vi "cRIO_8maze_controls_v3_nodoors.vi"() -> ()   [LabVIEW 2019]
panel:
  in  "Servo wait (ms)":u32=1000
  in  "Servo enable":bool
  in  "NO LEDs":bool
  in  "servo2PWM_R":dbl=3.4 format="%#_13g"
  in  "PWM initial":dbl[](array[numeric])=[9.5, 8.1, 5.1, 5.6]
  in  "MDServoPWM_R":dbl[](array[numeric])=[5.2, 5.45]
  in  "MDServoPWM_L":dbl[](array[numeric])=[5.2, 5.45]
  in  "No Milk":bool
  in  "Repeat sound":bool
  in  "Initialize":bool=TRUE
  in  "Air puff time":u32=1000
  in  "MD time (ms)":i32=3000
  out "Direction array":bool[](array[boolean])=[TRUE, FALSE, FALSE, TRUE, FALSE, TRUE, TRUE, FALSE, TRUE, FALSE, FALSE, TRUE, FALSE, TRUE, FALSE, FALSE, TRUE, FALSE, TRUE, TRUE, FALSE, TRUE, FALSE, FALSE, TRUE, FALSE, TRUE, TRUE, FALSE, TRUE, FALSE, FALSE, TRUE, FALSE, TRUE, TRUE, FALSE, TRUE, FALSE, FALSE, TRUE, FALSE, TRUE, TRUE, FALSE, TRUE, FALSE, FALSE, TRUE]
  out "Seq update":i32
  in  "Loop seq.":dbl
  out "All BBR":bool
  out "BB3_R":bool
  out "BB2_R":bool
  out "BB1_L":bool
  out "All BBL":bool
  out "BB3_L":bool
  out "BB2_L":bool
  out "BB1_R":bool
  out "Right":bool=TRUE
  in  "Sound":bool
  in  "AIR":bool
  out "Left":bool=TRUE
  in  "MD_R":bool
  in  "MD_L":bool
  in  "LED_R":bool
  in  "LED_L":bool
  in  "PWM rate":dbl[](array[numeric])=[0.1, 0.1, 0.1, 0.1]
  out "appended array":bool[](array[boolean])
  in  "PWM positions":dbl[](array[numeric])=[4.5, 3.4, 5.1, 5.8]
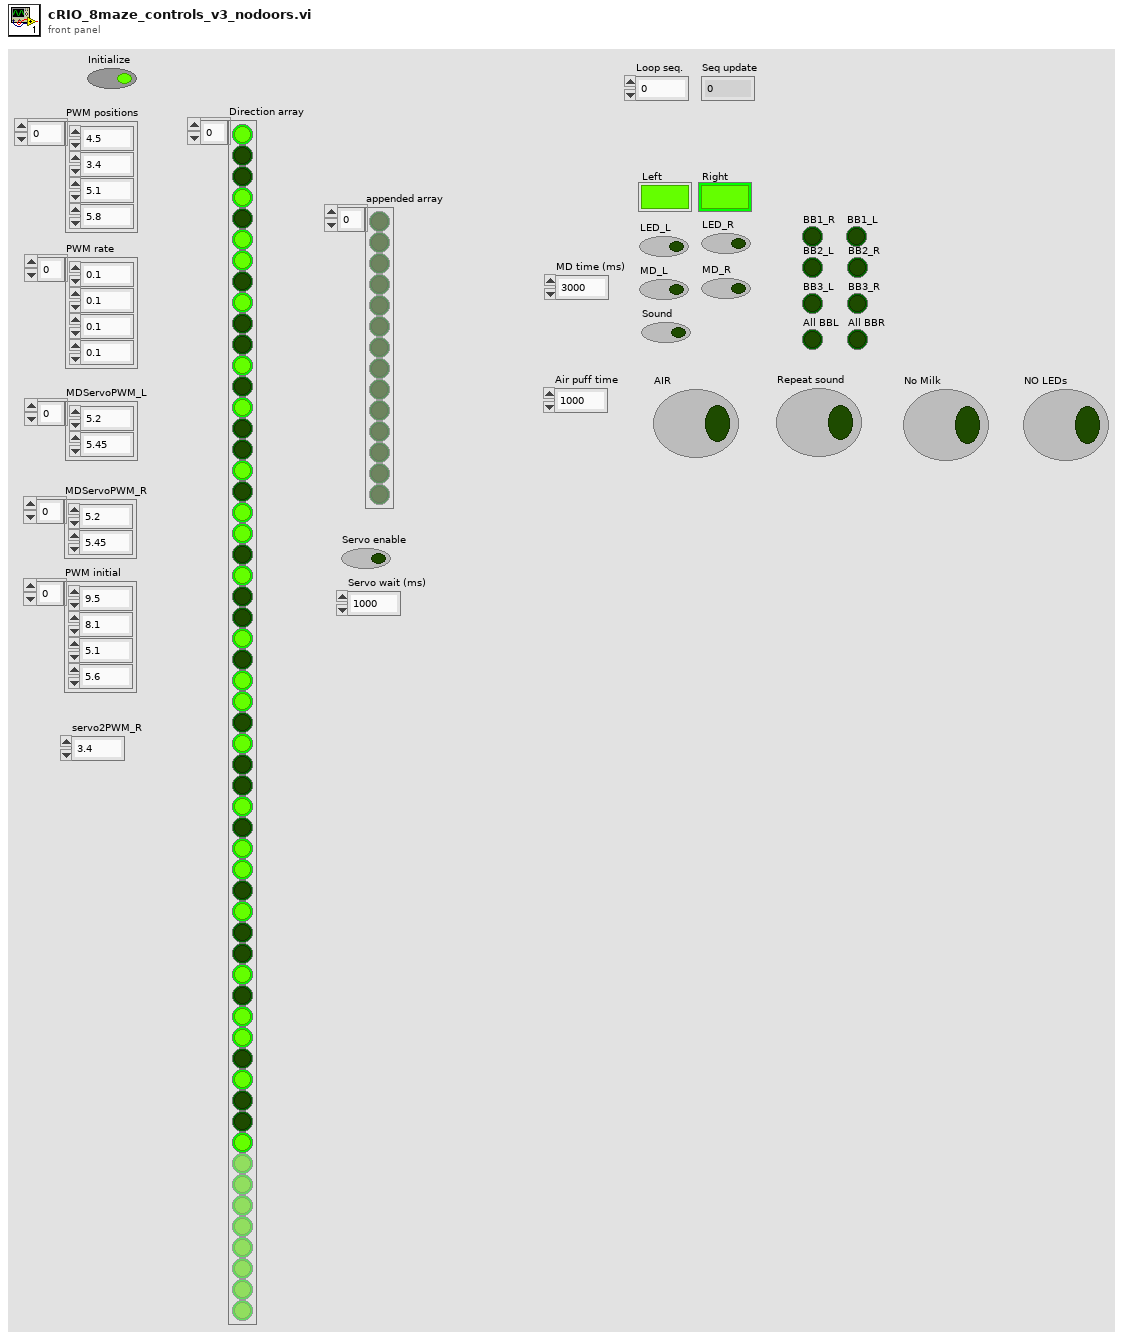
[diagram p1: front panel]
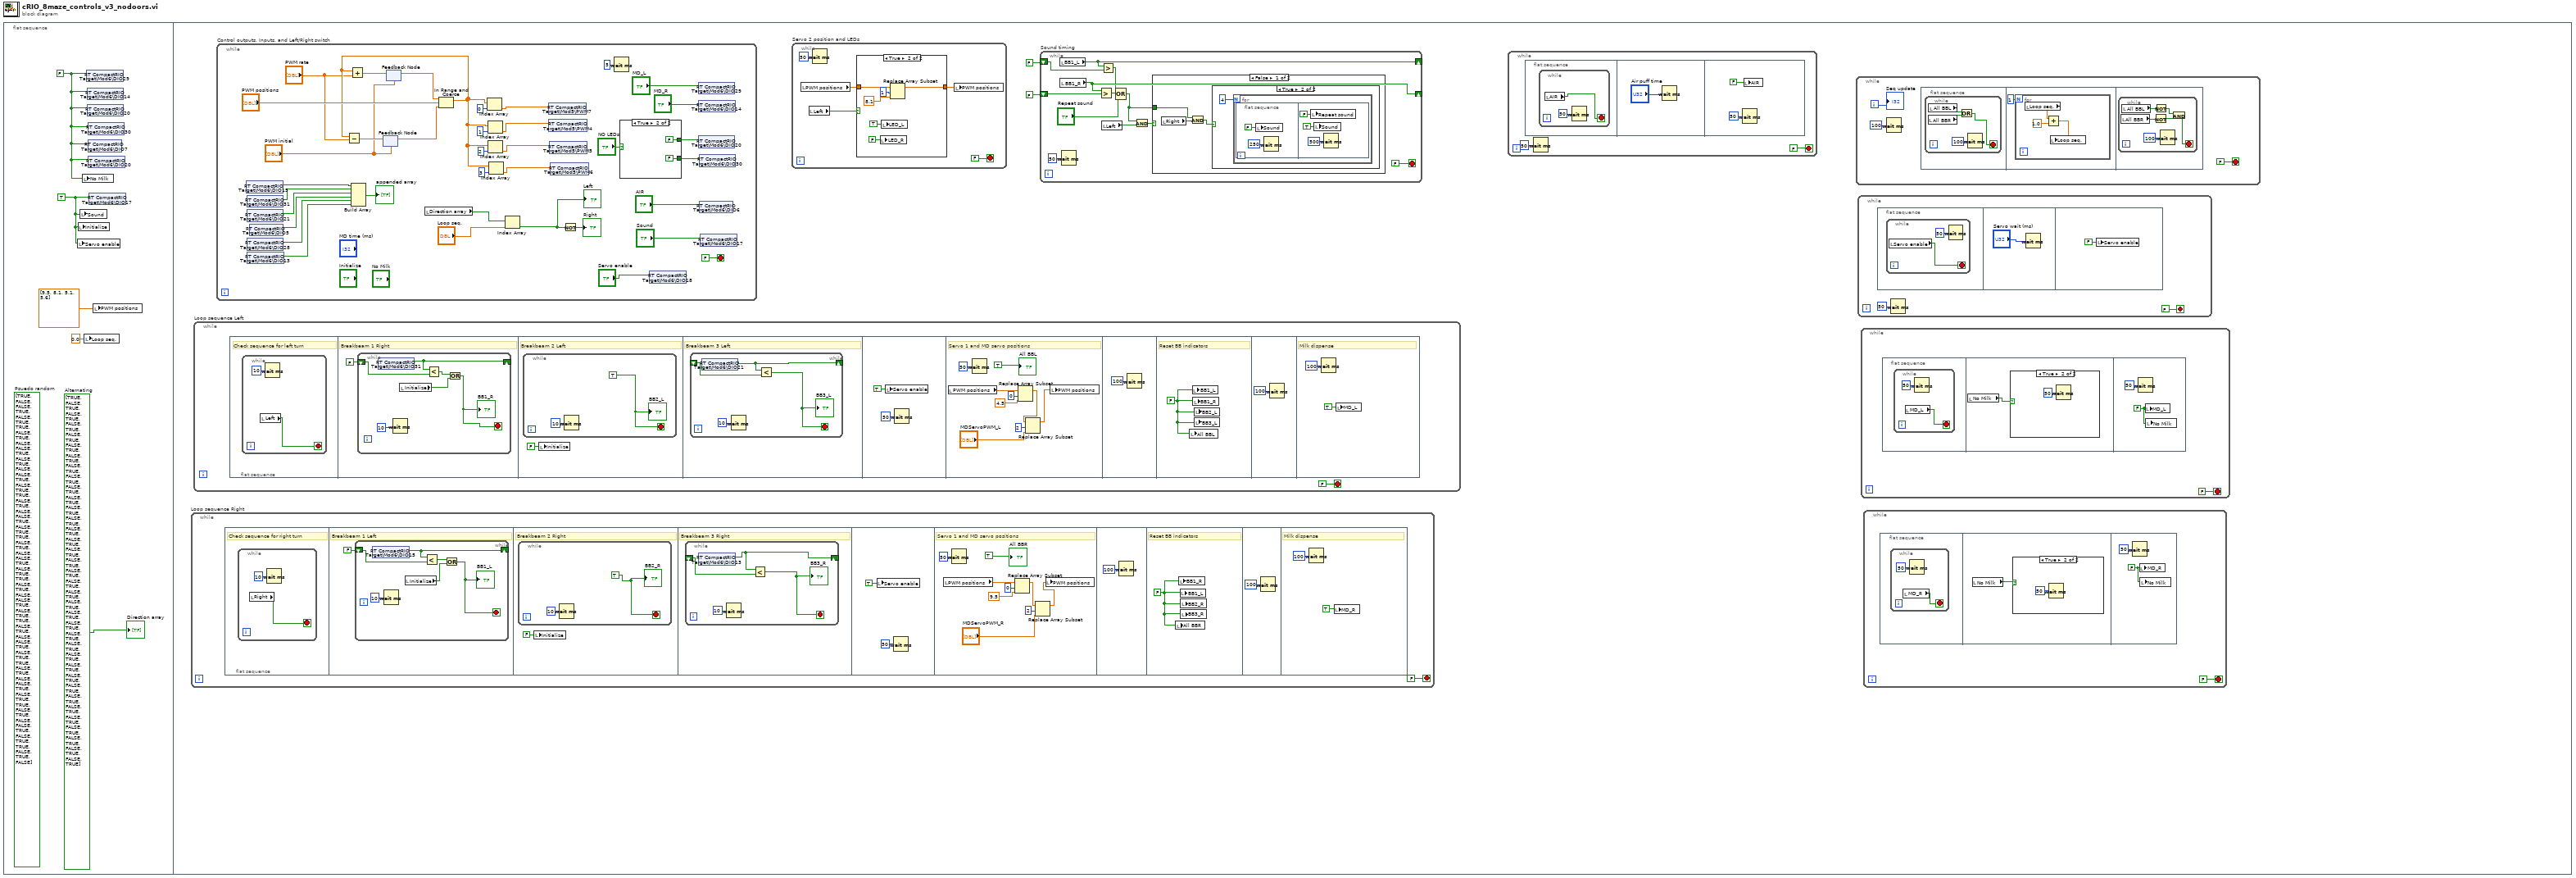
[diagram p0: block diagram]
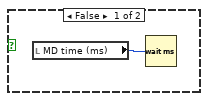
[diagram p2: hidden frame]
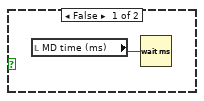
[diagram p3: hidden frame]
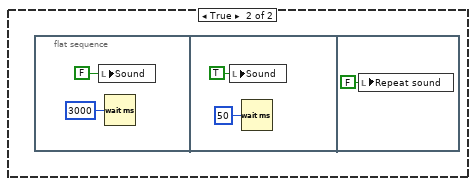
[diagram p5: hidden frame]
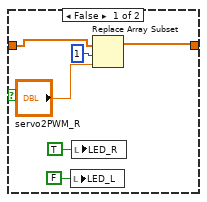
[diagram p6: hidden frame]
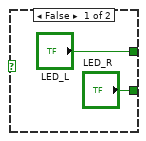
[diagram p7: hidden frame]
diagram:
  n1 = flat-sequence {
    frame #0 {
      w3 = bool[] [TRUE, FALSE, TRUE, FALSE, TRUE, FALSE, TRUE, FALSE, TRUE, FALSE, TRUE, FALSE, TRUE, FALSE, TRUE, FALSE, TRUE, FALSE, TRUE, FALSE, TRUE, FALSE, TRUE, FALSE, TRUE, FALSE, TRUE, FALSE, TRUE, FALSE, TRUE, FALSE, TRUE, FALSE, TRUE, FALSE, TRUE, FALSE, TRUE, FALSE, TRUE, FALSE, TRUE, FALSE, TRUE, FALSE, TRUE, FALSE, TRUE, FALSE, TRUE, FALSE, TRUE, FALSE, TRUE, FALSE, TRUE, FALSE, TRUE, FALSE, TRUE, FALSE, TRUE, FALSE, TRUE, FALSE, TRUE, FALSE, TRUE, FALSE, TRUE]  # Alternating
      (unwired) bool[] [TRUE, FALSE, FALSE, TRUE, FALSE, TRUE, TRUE, FALSE, TRUE, FALSE, FALSE, TRUE, FALSE, TRUE, FALSE, FALSE, TRUE, FALSE, TRUE, TRUE, FALSE, TRUE, FALSE, FALSE, TRUE, FALSE, TRUE, TRUE, FALSE, TRUE, FALSE, FALSE, TRUE, FALSE, TRUE, TRUE, FALSE, TRUE, FALSE, FALSE, TRUE, FALSE, TRUE, TRUE, FALSE, TRUE, FALSE, FALSE, TRUE, FALSE, TRUE, TRUE, FALSE, TRUE, FALSE, FALSE, TRUE, FALSE, TRUE, TRUE, FALSE, TRUE, FALSE, FALSE, TRUE, FALSE, TRUE, TRUE, FALSE, TRUE, FALSE]  # Psuedo random
      w1 = TRUE
      w2 = FALSE
      n2 = local write "Servo enable"(w1) -> ()
      n3 = local write "Initialize"(w1) -> ()
      n4 = local write "Sound"(w1) -> ()
      n5 = local write "No Milk"(w2) -> ()
      n6 = local write "Loop seq."(0.0 ("Loop seq.")) -> ()
      n7 = shared-variable "RT CompactRIO Target\\Mod6\\DIO29"(w2) -> ()  [unwired: 1 in, 1 out]
      n8 = shared-variable "RT CompactRIO Target\\Mod6\\DIO14"(w2) -> ()  [unwired: 1 in, 1 out]
      n9 = shared-variable "RT CompactRIO Target\\Mod6\\DIO20"(w2) -> ()  [unwired: 1 in, 1 out]
      n10 = shared-variable "RT CompactRIO Target\\Mod6\\DIO30"(w2) -> ()  [unwired: 1 in, 1 out]
      n11 = shared-variable "RT CompactRIO Target\\Mod6\\DIO7"(w2) -> ()  [unwired: 1 in, 1 out]
      n12 = shared-variable "RT CompactRIO Target\\Mod6\\DIO20"(w2) -> ()  [unwired: 1 in, 1 out]
      n13 = shared-variable "RT CompactRIO Target\\Mod6\\DIO17"(w1) -> ()  [unwired: 1 in, 1 out]
      n14 = local write "PWM positions"(dbl[] [9.5, 8.1, 5.1, 5.6]) -> ()
      "Direction array" <- w3
    }
    frame #1 {
      n15 = while "Loop sequence Right" {
        stop <- FALSE stop-if-true
        n16 = flat-sequence {
          frame #0 {
            # "Check sequence for right turn"
            n17 = while {
              stop <- w82 stop-if-true
              n18 = local read "Right"() -> (w82:bool)
              n19 = Wait (ms)(milliseconds to wait=u32 10) -> ()  [unwired: 1 out]
            }
          }
          frame #1 {
            # "Breakbeam 1 Left"
            n20 = while {
              shift-right: [w85] -> _
              shift-left: FALSE -> [w89]
              stop <- w84 stop-if-true
              n21 = shared-variable "RT CompactRIO Target\\Mod6\\DIO15"() -> (w85:bool)  [unwired: 1 in, 1 out]
              n22 = Wait (ms)(milliseconds to wait=u32 10) -> ()  [unwired: 1 out]
              n23 = local read "Initialize"() -> (w86:bool)
              n24 = Less?(x=w85, y=w89) -> (x < y?=w87:bool)
              n25 = Or(x=w87, y=w86) -> (x .or. y?=w84:bool)
              "BB1_L" <- w84
            }
          }
          frame #2 {
            # "Breakbeam 2 Right"
            n26 = while {
              stop <- w91 stop-if-true
              w91 = TRUE
              n27 = Wait (ms)(milliseconds to wait=u32 10) -> ()  [unwired: 1 out]
              "BB2_R" <- w91
            }
            n28 = local write "Initialize"(FALSE ("Initialize")) -> ()
          }
          frame #3 {
            # "Breakbeam 3 Right"
            n29 = while {
              shift-right: [w94] -> _
              shift-left: _ -> [w96]
              stop <- w93 stop-if-true
              n30 = shared-variable "RT CompactRIO Target\\Mod6\\DIO13"() -> (w94:bool)  [unwired: 1 in, 1 out]
              n31 = Wait (ms)(milliseconds to wait=u32 10) -> ()  [unwired: 1 out]
              n32 = Less?(x=w94, y=w96) -> (x < y?=w93:bool)
              "BB3_R" <- w93
            }
          }
          frame #4 {
            n33 = local write "Servo enable"(TRUE ("Servo enable")) -> ()
            n34 = Wait (ms)(milliseconds to wait=u32 50) -> ()  [unwired: 1 out]
          }
          frame #5 {
            # "Servo 1 and MD servo positions"
            n35 = local read "PWM positions"() -> (w105:dbl[])
            n36 = Wait (ms)(milliseconds to wait=u32 50) -> ()  [unwired: 1 out]
            n37 = Replace Array Subset(array=w105, new element=9.5 ("new element/subarray"), index=0) -> (w100:dbl[])
            n38 = Replace Array Subset(array=w100, new element="MDServoPWM_R", index=2) -> (w99:dbl[])
            n39 = local write "PWM positions"(w99) -> ()
            "All BBR" <- TRUE
          }
          frame #6 {
            n40 = Wait (ms)(milliseconds to wait=u32 100) -> ()  [unwired: 1 out]
          }
          frame #7 {
            w109 = FALSE
            # "Reset BB indicators"
            n41 = local write "All BBR"(w109) -> ()
            n42 = local write "BB1_R"(w109) -> ()
            n43 = local write "BB1_L"(w109) -> ()
            n44 = local write "BB2_R"(w109) -> ()
            n45 = local write "BB3_R"(w109) -> ()
          }
          frame #8 {
            n46 = Wait (ms)(milliseconds to wait=u32 100) -> ()  [unwired: 1 out]
          }
          frame #9 {
            # "Milk dispense"
            n47 = Wait (ms)(milliseconds to wait=u32 100) -> ()  [unwired: 1 out]
            n48 = local write "MD_R"(TRUE ("MD_R")) -> ()
          }
        }
      }
      n49 = while "Loop sequence Left" {
        stop <- FALSE stop-if-true
        n50 = flat-sequence {
          frame #0 {
            # "Check sequence for left turn"
            n51 = while {
              stop <- w132 stop-if-true
              n52 = local read "Left"() -> (w132:bool)
              n53 = Wait (ms)(milliseconds to wait=u32 10) -> ()  [unwired: 1 out]
            }
          }
          frame #1 {
            # "Breakbeam 1 Right"
            n54 = while {
              shift-right: [w134] -> _
              shift-left: FALSE -> [w139]
              stop <- w135 stop-if-true
              n55 = shared-variable "RT CompactRIO Target\\Mod6\\DIO31"() -> (w134:bool)  [unwired: 1 in, 1 out]
              n56 = Wait (ms)(milliseconds to wait=u32 10) -> ()  [unwired: 1 out]
              n57 = local read "Initialize"() -> (w136:bool)
              n58 = Less?(x=w134, y=w139) -> (x < y?=w137:bool)
              n59 = Or(x=w137, y=w136) -> (x .or. y?=w135:bool)
              "BB1_R" <- w135
            }
          }
          frame #2 {
            # "Breakbeam 2 Left"
            n60 = while {
              stop <- w141 stop-if-true
              w141 = TRUE
              n61 = Wait (ms)(milliseconds to wait=u32 10) -> ()  [unwired: 1 out]
              "BB2_L" <- w141
            }
            n62 = local write "Initialize"(FALSE ("Initialize")) -> ()
          }
          frame #3 {
            # "Breakbeam 3 Left"
            n63 = while {
              shift-right: [w144] -> _
              shift-left: _ -> [w146]
              stop <- w143 stop-if-true
              n64 = shared-variable "RT CompactRIO Target\\Mod6\\DIO21"() -> (w144:bool)  [unwired: 1 in, 1 out]
              n65 = Wait (ms)(milliseconds to wait=u32 10) -> ()  [unwired: 1 out]
              n66 = Less?(x=w144, y=w146) -> (x < y?=w143:bool)
              "BB3_L" <- w143
            }
          }
          frame #4 {
            n67 = local write "Servo enable"(TRUE ("Servo enable")) -> ()
            n68 = Wait (ms)(milliseconds to wait=u32 50) -> ()  [unwired: 1 out]
          }
          frame #5 {
            # "Servo 1 and MD servo positions"
            n69 = local read "PWM positions"() -> (w155:dbl[])
            n70 = Wait (ms)(milliseconds to wait=u32 50) -> ()  [unwired: 1 out]
            n71 = Replace Array Subset(array=w155, new element=4.5 ("new element/subarray"), index=0) -> (w150:dbl[])
            n72 = Replace Array Subset(array=w150, new element="MDServoPWM_L", index=2) -> (w149:dbl[])
            n73 = local write "PWM positions"(w149) -> ()
            "All BBL" <- TRUE
          }
          frame #6 {
            n74 = Wait (ms)(milliseconds to wait=u32 100) -> ()  [unwired: 1 out]
          }
          frame #7 {
            w159 = FALSE
            # "Reset BB indicators"
            n75 = local write "All BBL"(w159) -> ()
            n76 = local write "BB1_L"(w159) -> ()
            n77 = local write "BB1_R"(w159) -> ()
            n78 = local write "BB2_L"(w159) -> ()
            n79 = local write "BB3_L"(w159) -> ()
          }
          frame #8 {
            n80 = Wait (ms)(milliseconds to wait=u32 100) -> ()  [unwired: 1 out]
          }
          frame #9 {
            # "Milk dispense"
            n81 = Wait (ms)(milliseconds to wait=u32 100) -> ()  [unwired: 1 out]
            n82 = local write "MD_L"(TRUE ("MD_L")) -> ()
          }
        }
      }
      n83 = while "Control outputs, Inputs, and Left/Right switch" {
        stop <- FALSE stop-if-true
        n84 = shared-variable "RT CompactRIO Target\\Mod6\\DIO15"() -> (w179:bool)  [unwired: 1 in, 1 out]
        n85 = shared-variable "RT CompactRIO Target\\Mod6\\DIO31"() -> (w173:bool)  [unwired: 1 in, 1 out]
        n86 = shared-variable "RT CompactRIO Target\\Mod6\\DIO21"() -> (w174:bool)  [unwired: 1 in, 1 out]
        n87 = shared-variable "RT CompactRIO Target\\Mod6\\DIO28"() -> (w176:bool)  [unwired: 1 in, 1 out]
        n88 = shared-variable "RT CompactRIO Target\\Mod6\\DIO13"() -> (w177:bool)  [unwired: 1 in, 1 out]
        n89 = shared-variable "RT CompactRIO Target\\Mod6\\DIO5"() -> (w175:bool)  [unwired: 1 in, 1 out]
        n90 = Build Array(w179, w173, w174, w175, w176, w177) -> (→"appended array":bool[])
        n91 = feedback #1("PWM initial") -> (w186:dbl[])
        n92 = feedback #2("PWM initial") -> (w189:dbl[])
        n93 = local read "Direction array"() -> (w166:bool[])
        n94 = In Range and Coerce(upper limit=w189, x="PWM positions", lower limit=w186) -> (coerced(x)=w188:dbl[])  [unwired: 1 out]
        n95 = Subtract(x=w188, y="PWM rate") -> (x-y=w187:dbl[])
        n96 = Add(x=w188, y="PWM rate") -> (x+y=w190:dbl[])
        n97 = feedback-in #1(w187) -> ()
        n98 = feedback-in #2(w190) -> ()
        n99 = Index Array(array=w188, index=0) -> (element=w169:dbl)
        n100 = Index Array(array=w188, index=1) -> (element=w168:dbl)
        n101 = Index Array(array=w188, index=2) -> (element=w198:dbl)
        n102 = Index Array(array=w188, index=3) -> (element=w199:dbl)
        n103 = Index Array(array=w166, index="Loop seq.") -> (element=w167:bool)
        "Left" <- w167
        n104 = shared-variable "RT CompactRIO Target\\Mod5\\PWM7"(w169) -> ()  [unwired: 1 in, 1 out]
        n105 = shared-variable "RT CompactRIO Target\\Mod5\\PWM4"(w168) -> ()  [unwired: 1 in, 1 out]
        n106 = shared-variable "RT CompactRIO Target\\Mod5\\PWM5"(w198) -> ()  [unwired: 1 in, 1 out]
        n107 = shared-variable "RT CompactRIO Target\\Mod5\\PWM6"(w199) -> ()  [unwired: 1 in, 1 out]
        n108 = Not(x=w167) -> (.not. x?=→"Right":bool)
        n109 = Wait (ms)(milliseconds to wait=u32 5) -> ()  [unwired: 1 out]
        n110 = case shown="True" "NO LEDs" {
          tunnel: ["LED_R" FALSE ("LED_R")] -> w181
          tunnel: ["LED_L" FALSE ("LED_L")] -> w180
          frame False {
          }
          frame True {
          }
        }
        n111 = shared-variable "RT CompactRIO Target\\Mod6\\DIO18"("Servo enable") -> ()  [unwired: 1 in, 1 out]
        n112 = shared-variable "RT CompactRIO Target\\Mod6\\DIO29"("MD_L") -> ()  [unwired: 1 in, 1 out]
        n113 = shared-variable "RT CompactRIO Target\\Mod6\\DIO20"(w180) -> ()  [unwired: 1 in, 1 out]
        n114 = shared-variable "RT CompactRIO Target\\Mod6\\DIO14"("MD_R") -> ()  [unwired: 1 in, 1 out]
        n115 = shared-variable "RT CompactRIO Target\\Mod6\\DIO30"(w181) -> ()  [unwired: 1 in, 1 out]
        n116 = shared-variable "RT CompactRIO Target\\Mod6\\DIO6"("AIR") -> ()  [unwired: 1 in, 1 out]
        n117 = shared-variable "RT CompactRIO Target\\Mod6\\DIO17"("Sound") -> ()  [unwired: 1 in, 1 out]
      }
      n118 = while "Servo 2 position and LEDs" {
        stop <- FALSE stop-if-true
        n119 = local read "PWM positions"() -> (w115:dbl[])
        n120 = local read "Left"() -> (w116:bool)
        n121 = Wait (ms)(milliseconds to wait=u32 50) -> ()  [unwired: 1 out]
        n122 = case shown="True" w116 {
          tunnel: w115 -> [w121 w127]
          tunnel: [w120 w126] -> w114
          frame False {
            n123 = local write "LED_L"(FALSE ("LED_L")) -> ()
            n124 = local write "LED_R"(TRUE ("LED_R")) -> ()
            n125 = Replace Array Subset(array=w121, new element="servo2PWM_R", index=1) -> (w120:dbl[])
          }
          frame True {
            n126 = local write "LED_R"(FALSE ("LED_R")) -> ()
            n127 = local write "LED_L"(TRUE ("LED_L")) -> ()
            n128 = Replace Array Subset(array=w127, new element=8.1 ("new element/subarray"), index=1) -> (w126:dbl[])
          }
        }
        n129 = local write "PWM positions"(w114) -> ()
      }
      n130 = while "Sound timing" {
        shift-right: [w47] -> _
        shift-left: FALSE ("BB1_L") -> [w46]
        shift-right: [w41] -> _
        shift-left: FALSE ("BB1_R") -> [w42]
        stop <- FALSE stop-if-true
        n131 = local read "BB1_L"() -> (w41:bool)
        n132 = local read "BB1_R"() -> (w47:bool)
        n133 = Wait (ms)(milliseconds to wait=u32 50) -> ()  [unwired: 1 out]
        n134 = Greater?(x=w47, y=w46) -> (0:w40:bool)
        n135 = Greater?(x=w41, y=w42) -> (0:w39:bool)
        n136 = local read "Left"() -> (w45:bool)
        n137 = Compound Arithmetic op=OR(w39, w40, "Repeat sound") -> (w38:bool)
        n138 = And(x=w38, y=w45) -> (x .and. y?=w44:bool)
        n139 = case shown="False" w44 {
          tunnel: w38 -> [w51 _]
          frame False {
            n140 = local read "Right"() -> (w50:bool)
            n141 = And(x=w51, y=w50) -> (x .and. y?=w49:bool)
            n142 = case shown="True" w49 {
              frame False {
              }
              frame True {
                n143 = for {
                  N: 4 -> [_]
                  n144 = flat-sequence {
                    frame #0 {
                      n145 = local write "Sound"(FALSE ("Sound")) -> ()
                      n146 = Wait (ms)(milliseconds to wait=u32 250) -> ()  [unwired: 1 out]
                    }
                    frame #1 {
                      n147 = local write "Repeat sound"(FALSE ("Repeat sound")) -> ()
                      n148 = local write "Sound"(TRUE ("Sound")) -> ()
                      n149 = Wait (ms)(milliseconds to wait=u32 500) -> ()  [unwired: 1 out]
                    }
                  }
                }
              }
            }
          }
          frame True {
            n150 = flat-sequence {
              frame #0 {
                n151 = local write "Sound"(FALSE ("Sound")) -> ()
                n152 = Wait (ms)(milliseconds to wait=u32 3000) -> ()  [unwired: 1 out]
              }
              frame #1 {
                n153 = local write "Sound"(TRUE ("Sound")) -> ()
                n154 = Wait (ms)(milliseconds to wait=u32 50) -> ()  [unwired: 1 out]
              }
              frame #2 {
                n155 = local write "Repeat sound"(FALSE ("Repeat sound")) -> ()
              }
            }
          }
        }
      }
      n156 = while {
        stop <- FALSE stop-if-true
        n157 = flat-sequence {
          frame #0 {
            n158 = while {
              stop <- w32 stop-if-true
              n159 = local read "AIR"() -> (w32:bool)
              n160 = Wait (ms)(milliseconds to wait=u32 50) -> ()  [unwired: 1 out]
            }
          }
          frame #1 {
            n161 = Wait (ms)(milliseconds to wait="Air puff time") -> ()  [unwired: 1 out]
          }
          frame #2 {
            n162 = Wait (ms)(milliseconds to wait=u32 50) -> ()  [unwired: 1 out]
            n163 = local write "AIR"(FALSE ("AIR_L")) -> ()
          }
        }
        n164 = Wait (ms)(milliseconds to wait=u32 50) -> ()  [unwired: 1 out]
      }
      n165 = while {
        i -> [w63]
        stop <- FALSE stop-if-true
        n166 = Wait (ms)(milliseconds to wait=u32 100) -> ()  [unwired: 1 out]
        n167 = flat-sequence {
          frame #0 {
            n168 = while {
              stop <- w66 stop-if-true
              n169 = local read "All BBR"() -> (w67:bool)
              n170 = local read "All BBL"() -> (w68:bool)
              n171 = Or(x=w68, y=w67) -> (x .or. y?=w66:bool)
              n172 = Wait (ms)(milliseconds to wait=u32 100) -> ()  [unwired: 1 out]
            }
          }
          frame #1 {
            n173 = for {
              N: 1 -> [_]
              n174 = local read "Loop seq."() -> (w73:dbl)
              n175 = Add(x=w73, y=1.0) -> (x+y=w71:dbl)
              n176 = local write "Loop seq."(w71) -> ()
            }
          }
          frame #2 {
            n177 = while {
              stop <- w74 stop-if-true
              n178 = local read "All BBR"() -> (w77:bool)
              n179 = local read "All BBL"() -> (w78:bool)
              n180 = Not(x=w77) -> (.not. x?=w75:bool)
              n181 = Not(x=w78) -> (.not. x?=w76:bool)
              n182 = Wait (ms)(milliseconds to wait=u32 100) -> ()  [unwired: 1 out]
              n183 = And(x=w76, y=w75) -> (x .and. y?=w74:bool)
            }
          }
        }
        "Seq update" <- w63
      }
      n184 = while {
        stop <- FALSE stop-if-true
        n185 = flat-sequence {
          frame #0 {
            n186 = while {
              stop <- w11 stop-if-true
              n187 = local read "Servo enable"() -> (w11:bool)
              n188 = Wait (ms)(milliseconds to wait=u32 50) -> ()  [unwired: 1 out]
            }
          }
          frame #1 {
            n189 = Wait (ms)(milliseconds to wait="Servo wait (ms)") -> ()  [unwired: 1 out]
          }
          frame #2 {
            n190 = local write "Servo enable"(FALSE ("Servo enable")) -> ()
          }
        }
        n191 = Wait (ms)(milliseconds to wait=u32 50) -> ()  [unwired: 1 out]
      }
      n192 = while {
        stop <- FALSE stop-if-true
        n193 = flat-sequence {
          frame #0 {
            n194 = while {
              stop <- w24 stop-if-true
              n195 = local read "MD_L"() -> (w24:bool)
              n196 = Wait (ms)(milliseconds to wait=u32 50) -> ()  [unwired: 1 out]
            }
          }
          frame #1 {
            n197 = local read "No Milk"() -> (w25:bool)
            n198 = case shown="True" w25 {
              frame False {
                n199 = local read "MD time (ms)"() -> (w26:i32)
                n200 = Wait (ms)(milliseconds to wait=w26) -> ()  [unwired: 1 out]
              }
              frame True {
                n201 = Wait (ms)(milliseconds to wait=u32 50) -> ()  [unwired: 1 out]
              }
            }
          }
          frame #2 {
            w28 = FALSE ("MD_L")
            n202 = Wait (ms)(milliseconds to wait=u32 50) -> ()  [unwired: 1 out]
            n203 = local write "MD_L"(w28) -> ()
            n204 = local write "No Milk"(w28) -> ()
          }
        }
      }
      n205 = while {
        stop <- FALSE stop-if-true
        n206 = flat-sequence {
          frame #0 {
            n207 = while {
              stop <- w16 stop-if-true
              n208 = local read "MD_R"() -> (w16:bool)
              n209 = Wait (ms)(milliseconds to wait=u32 50) -> ()  [unwired: 1 out]
            }
          }
          frame #1 {
            n210 = local read "No Milk"() -> (w17:bool)
            n211 = case shown="True" w17 {
              frame False {
                n212 = local read "MD time (ms)"() -> (w18:i32)
                n213 = Wait (ms)(milliseconds to wait=w18) -> ()  [unwired: 1 out]
              }
              frame True {
                n214 = Wait (ms)(milliseconds to wait=u32 50) -> ()  [unwired: 1 out]
              }
            }
          }
          frame #2 {
            w20 = FALSE ("MD_R")
            n215 = Wait (ms)(milliseconds to wait=u32 50) -> ()  [unwired: 1 out]
            n216 = local write "MD_R"(w20) -> ()
            n217 = local write "No Milk"(w20) -> ()
          }
        }
      }
    }
  }
